vi "Count Boolean Change.vi"(1 "reset":bool, 2 "In":bool) -> (0 "Out":dbl)   [LabVIEW 2019]
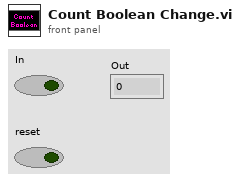
[diagram p1: front panel]
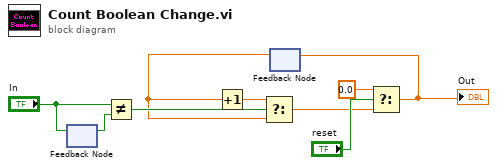
[diagram p0: block diagram]
diagram:
  n1 = feedback #1() -> (w5:bool)  [unwired: 1 in]
  n2 = feedback-in #1("In") -> ()
  n3 = Not Equal?(x="In", y=w5) -> (x != y?=w8:bool)
  n4 = feedback #2() -> (w7:dbl)  [unwired: 1 in]
  n5 = Increment(x=w7) -> (x+1=w9:dbl)
  n6 = Select(t=w9, s=w8, f=w7) -> (s? t:f=w1:dbl)
  n7 = Select(t=0.0, s="reset", f=w1) -> (s? t:f=w4:dbl)
  "Out" <- w4
  n8 = feedback-in #2(w4) -> ()
